vi "Begin by Reference.vi"(8 "Error In":errorcluster, 10 "Msgpack Data":u8[](array[numeric]), 11 "Reader In":refnum<data-value>) -> (0 "Error Out":errorcluster, 3 "Reader Out":refnum<data-value>)   [LabVIEW 2019, in "LabPack.lvlib" / "Reader.lvclass"]
uses:
  Reader.lvclass
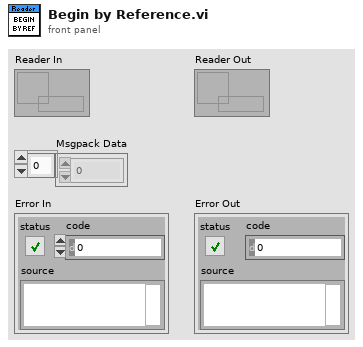
[diagram p1: front panel]
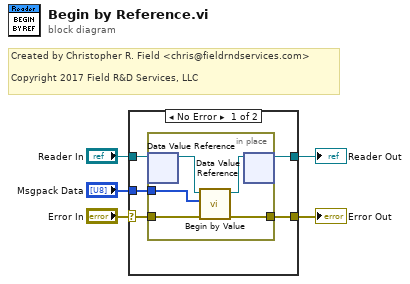
[diagram p0: block diagram]
diagram:
  # "Created by Christopher R. Field <chris@fieldrndservices.com>\n\nCopyright 2017 Field R&D Services, LLC"
  n1 = case shown="No Error" "Error In" {
    selector: "Error In" -> [w8 w16]
    tunnel: "Reader In" -> [w10 w17]
    tunnel: [w9 w17] -> w4
    tunnel: "Msgpack Data" -> [w7 _]
    tunnel: [w6 w16] -> w1
    frame No Error {
      n2 = in-place {
        in-place-border: w8 -> [w13]
        in-place-border: w7 -> [w12]
        in-place-border: [w11] -> w6
        n3 = in-place-dvr #1(w10) -> (w15:refnum<class "Reader.lvclass">)  [unwired: 1 out]
        n4 = call "Begin by Value.vi"("Error In"=w13, "Msgpack Data"=w12, "Reader In"=w15) -> ("Error Out"=w11:errorcluster, "Reader Out"=w14:refnum<class "Reader.lvclass">)  [unwired: 7 in]
        n5 = in-place-dvr #1(w14) -> (w9:refnum<data-value>)  [unwired: 1 out]
      }
    }
    frame Error {
    }
  }
  "Reader Out" <- w4
  "Error Out" <- w1
